vi "Autonomous Independent.vi"   [LabVIEW 2019]
doc: "This VI is called when autonomous begins, and will automatically be terminated when autonomous ends. You can carry out timed or sensor driven robot movement independently without needing to return to the caller."
uses:
  <vilib>/Rock Robotics/Network Tables/NT Read String.vi
  Encoder Recorder.lvlib
  Robot Global Data.vi
panel:
  # "Be sure to right-click and choose Data Operations>>Make Current Value default if you want to save the array values with the VI"
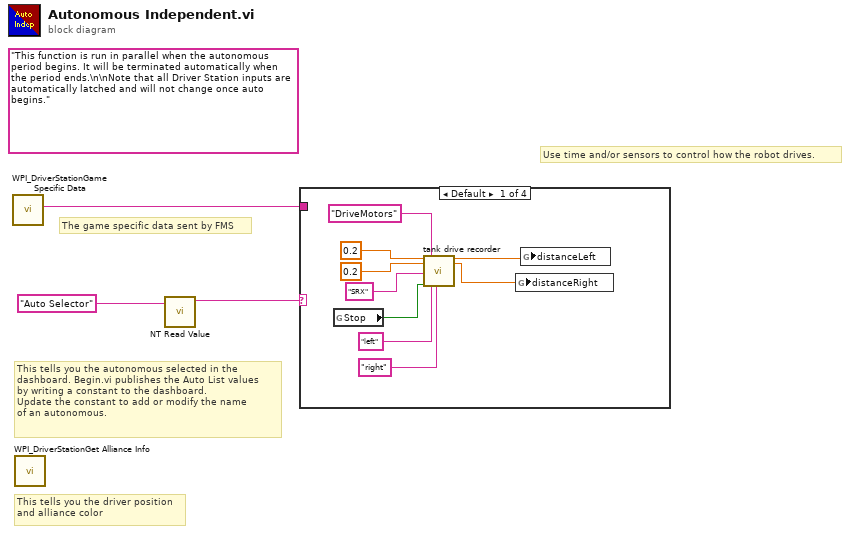
[diagram p0: block diagram]
diagram:
  (unwired) "This function is run in parallel when the autonomous period begins. It will be terminated automatically when the period ends.\n\nNote that all Driver Station inputs are automatically latched and will not change once auto begins."
  # "The game specific data sent by FMS"
  # "This tells you the autonomous selected in the \ndashboard. Begin.vi publishes the Auto List values\nby writing a constant to the dashboard.\nUpdate the constant to add or modify the name\nof an autonomous."
  # "Use time and/or sensors to control how the robot drives."
  # "This tells you the driver position\nand alliance color"
  n1 = call <vilib>:"WPI_DriverStationGame Specific Data.vi"() -> ("Game Specific Data"=w1:string)  [unwired: 11 in]
  n2 = call <vilib>:"WPI_DriverStationGet Alliance Info.vi"() -> ()  [unwired: 12 out]
  n3 = call-poly <vilib>:"NT Read Value.vi"("Name"="Auto Selector") -> ("String"=w2:string)  [unwired: 9 in, 1 out]
  n4 = case shown="Default" w2 {
    tunnel: w1 -> [_ _ _ _]
    frame Default {
      n5 = global read "Robot Global Data.vi" "Stop"() -> (w4:bool)
      n6 = call "tank drive recorder.vi"("leftSpeed"=0.2, "rightSpeed"=0.2, "motorController"="SRX", "stop"=w4, "driveMotors"="DriveMotors", "leftMotor"="left", "rightMotor"="right") -> ("distanceLeft"=w5:dbl, "distanceRight"=w6:dbl)  [unwired: 11 in]
      n7 = global write "Robot Global Data.vi" "distanceRight"(w6) -> ()
      n8 = global write "Robot Global Data.vi" "distanceLeft"(w5) -> ()
    }
    frame "Alternative 1" {
    }
    frame "Alternative 2" {
    }
    frame "Your Turn" {
    }
  }
